vi "inputToActivate.vi"(8 "error in (no error)":errorcluster, 9 "AviableSpec":u8[](array[numeric]), 10 "NumOfDevices":i32, 11 "SEDSpectrometer in":refnum<class "SEDSpectrometer.lvclass">) -> (0 "error out":errorcluster, 2 "InputActivate":u8[](array[numeric]), 3 "SEDSpectrometer out":refnum<class "SEDSpectrometer.lvclass">)   [LabVIEW 2016, in "SEDSpectrometer.lvclass"]
uses:
  SEDSpectrometer.lvclass
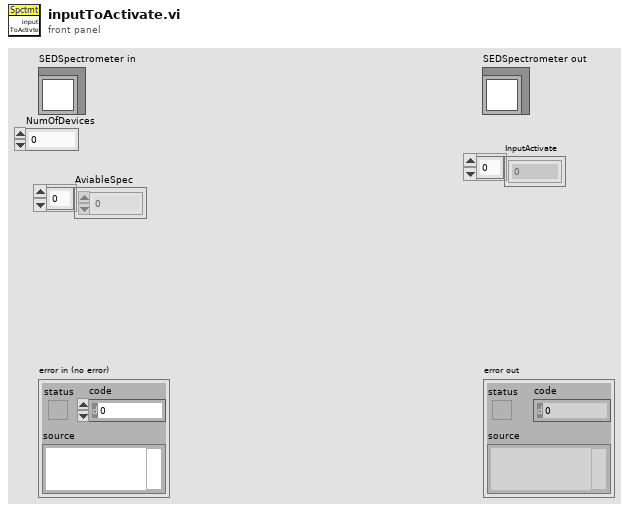
[diagram p1: front panel]
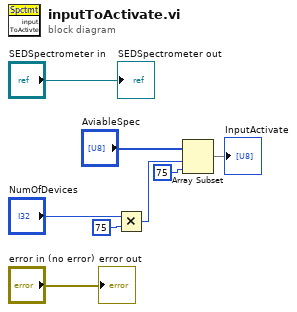
[diagram p0: block diagram]
diagram:
  n1 = Multiply(x="NumOfDevices", y=75 ("x")) -> (x*y=w4:i32)
  n2 = Array Subset(array="AviableSpec", index=w4, length=75 ("x")) -> (→"InputActivate":u8[])
  "error out" <- "error in (no error)"
  "SEDSpectrometer out" <- "SEDSpectrometer in"
